vi "Ball Align(SubVI).vi"(0 "Align X - t, Y - f":bool, 2 "accuracy":u32=100, 3 "x is in range":bool, 4 "y is in range":bool, 5 "L_PWM":dbl=0.3, 6 "R_PWM":dbl=0.3, 7 "curX":dbl, 8 "defY":dbl, 9 "curY":dbl, 14 "defX":dbl, 16 "RangeY":dbl, 18 "RangeX":dbl=20.0) -> (13 "x_is_in_range":bool, 15 "y_is_in_range":bool, 19 "Ready to Grab()":bool, 20 "Align_X-t,Y-f":bool, 22 "accuracy out":u32=100, 26 "L_PWM out":dbl, 27 "R_PWM out":dbl)   [LabVIEW 2017]
uses:
  <vilib>/myRIO/Instrument Drivers/Onboard IO/DIO/typedefs/DIO Reference.ctl
  <vilib>/myRIO/Common/Instrument Driver Framework/Utilities/typedefs/myRIO Generic Hardware Reference.ctl
  <vilib>/myRIO/Common/Instrument Driver Framework/Utilities/typedefs/Hardware Version Enum.ctl
  <vilib>/myRIO/Common/Instrument Driver Framework/Utilities/typedefs/myRIO v1.0 Reference.ctl
  <vilib>/myRIO/Common/Instrument Driver Framework/Utilities/typedefs/Generic FPGA Reference.ctl
  <vilib>/myRIO/Common/Instrument Driver Framework/myRIO v1.0/DIO/typedefs/DIO Channels List.ctl
  <vilib>/myRIO/Common/Instrument Driver Framework/myRIO v1.0/DIO/typedefs/DIO Channels Enum.ctl
  <vilib>/userdefined/High Color/nirio_resource_hc.ctl
  <vilib>/myRIO/Common/Instrument Driver Framework/Utilities/vis/Is FPGA Ref Available.vi
  <vilib>/myRIO/Common/Instrument Driver Framework/myRIO v1.0/DIO/vis/myRIO v1.1 Open DIO.vi
  <vilib>/myRIO/Instrument Drivers/Onboard IO/DIO/vis/Write.vi
  <vilib>/myRIO/Common/Instrument Driver Framework/Utilities/vis/Validate Channels.vi
  <vilib>/myRIO/Common/Instrument Driver Framework/myRIO v1.0/DIO/vis/myRIO v1.0 Reserve DIO.vi
  <vilib>/myRIO/Common/Instrument Driver Framework/myRIO v1.0/Resource Manager/vis/myRIO v1.0 Reserve Channel List.vi
  <vilib>/myRIO/Common/Instrument Driver Framework/myRIO v1.0/DIO/vis/myRIO v1.0 Build MUX Configuration DIO.vi
  <vilib>/myRIO/Common/Instrument Driver Framework/myRIO v1.0/Resource Manager/vis/myRIO v1.0 Reserve Channel.vi
  <vilib>/myRIO/Common/Instrument Driver Framework/myRIO v1.0/Resource Manager/vis/myRIO v1.0 Unreserve Channel.vi
  <vilib>/myRIO/Common/Instrument Driver Framework/myRIO v1.0/Resource Manager/vis/myRIO v1.0 Create Configuration List.vi
  <vilib>/myRIO/Common/Instrument Driver Framework/myRIO v1.0/Resource Manager/vis/myRIO v1.0 Build Mutex Name.vi
  <vilib>/Utility/VariantDataType/GetNumericInfo.vi
  <vilib>/Utility/error.llb/Error Cluster From Error Code.vi
  <vilib>/myRIO/Common/Instrument Driver Framework/myRIO v1.0/myRIO v1.1 Open.vi
  <vilib>/myRIO/Common/Instrument Driver Framework/Utilities/vis/IO Manager.vi
  <vilib>/myRIO/Common/Instrument Driver Framework/Utilities/vis/Configuration Manager.vi
  <vilib>/myRIO/Common/Instrument Driver Framework/myRIO v1.0/Resource Manager/vis/myRIO v1.0 Configure IO.vi
  <vilib>/myRIO/Common/Instrument Driver Framework/myRIO v1.0/myRIO v1.0 Close.vi
  <vilib>/myRIO/Common/Instrument Driver Framework/myRIO v1.0/DIO/vis/myRIO v1.0 Write DIO.vi
  <vilib>/myRIO/Express VI/Onboard IO/DO/DO Express VI.xnode
  <vilib>/myRIO/Instrument Drivers/Onboard IO/DIO/vis/myRIO DIO Open.xnode
  <vilib>/myRIO/Instrument Drivers/Onboard IO/DIO/DIO.lvlib
panel:
  out "DEF R_PWM":dbl
  out "DEF L_PWM":dbl
  in  "extra power":dbl=0.2 format="%#_13g"
  in  "range for boost":dbl=250.0
  out "offset":bool
  in  "M_offsetX":dbl=30.0
  in  "M_defY":dbl=250.0
  out "Right+":bool
  out "Left-":bool
  out "Left+":bool
  out "Right-":bool
  # "IN"
  # "OUT"
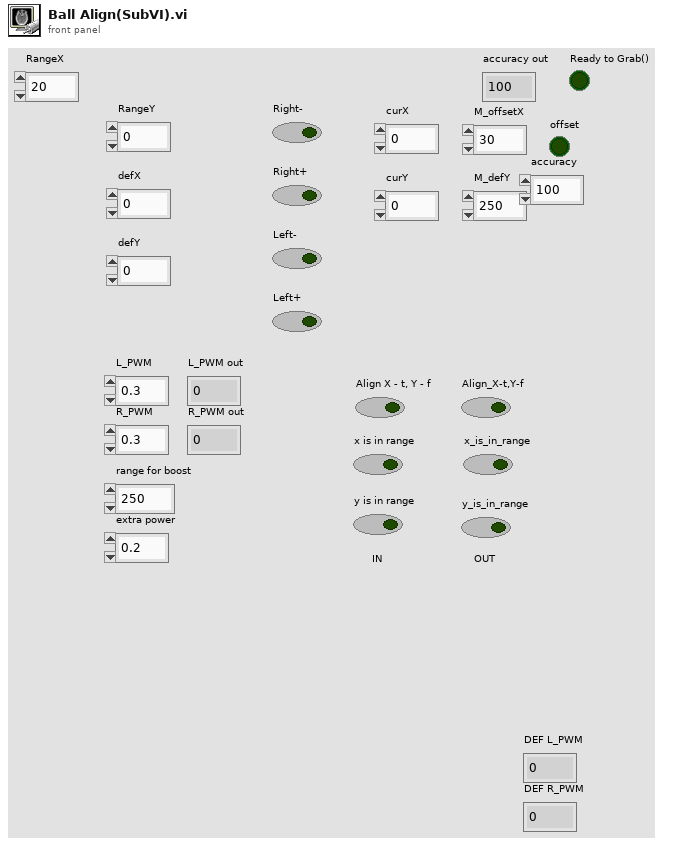
[diagram p1: front panel]
types:
  T1 = typedef "DIO.lvlib/DIO Reference.ctl" = cluster{"myRIO Reference":T2, "DIO Channels List":T6}
  T2 = typedef "myRIO Generic Hardware Reference.ctl" = cluster{"myRIO Model":T3, "myRIO Hardware Reference":T4}
  T3 = typedef "Hardware Version Enum.ctl" = enum16{"Unknown", "myRIO-1900", "myRIO-1950", "roboRIO", "NI ELVIS RIO CM"}
  T4 = typedef "myRIO v1.0 Reference.ctl" = cluster{"Generic FPGA Reference":T5, "Allow multiple opens":bool}
  T5 = typedef "Generic FPGA Reference.ctl" = refnum<k20>
  T6 = typedef "DIO Channels List.ctl" = T7[]
  T7 = typedef "DIO Channels Enum.ctl" = enum16{"Not Connected", "C/DIO0", "C/DIO1", "C/DIO2", "C/DIO3", "C/DIO4", "C/DIO5", "C/DIO6", "C/DIO7", "A/DIO0", "A/DIO1", "A/DIO2", "A/DIO3", "A/DIO4", "A/DIO5", "A/DIO6", "A/DIO7", "A/DIO8", "A/DIO9", "A/DIO10", "A/DIO11", "A/DIO12", "A/DIO13", "A/DIO14", "A/DIO15", "B/DIO0", "B/DIO1", "B/DIO2", "B/DIO3", "B/DIO4", "B/DIO5", "B/DIO6", "B/DIO7", "B/DIO8", "B/DIO9", "B/DIO10", "B/DIO11", "B/DIO12", "B/DIO13", "B/DIO14", "B/DIO15", "LED0", "LED1", "LED2", "LED3", "Button0", "DIO/DIO0", "DIO/DIO1", "DIO/DIO2", "DIO/DIO3", "DIO/DIO4", "DIO/DIO5", "DIO/DIO6", "DIO/DIO7", "DIO/DIO8", "DIO/DIO9", "SPI/CS0", "SPI/CS1", "SPI/CS2", "SPI/CS3", "LED RADIO (Green)", "LED RADIO (Red)", "LED COMM (Green)", "LED COMM (Red)", "LED MODE (Green)", "LED MODE (Red)"}
  T8 = typedef "nirio_resource_hc.ctl" = tag
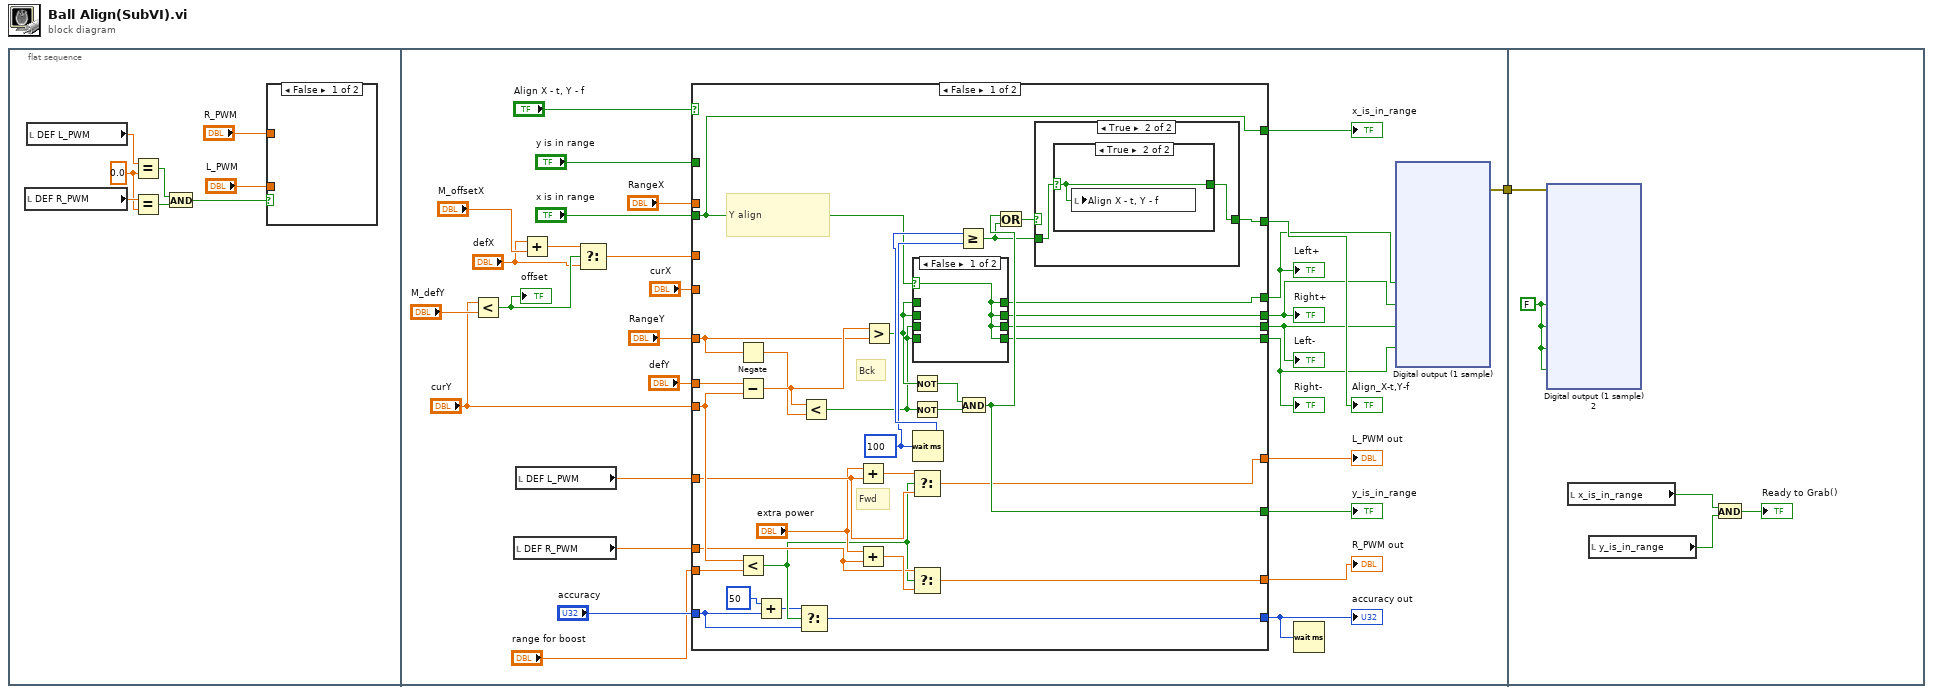
[diagram p0: block diagram]
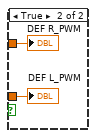
[diagram p2: hidden frame]
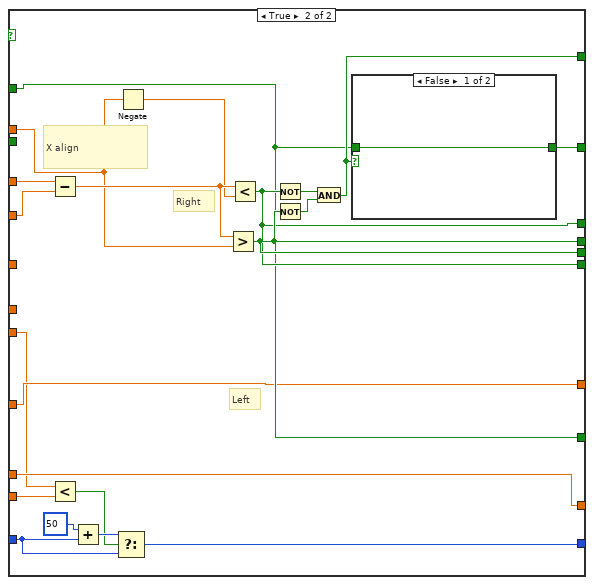
[diagram p6: hidden frame]
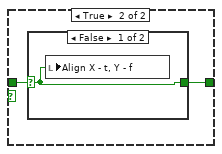
[diagram p7: hidden frame]
diagram:
  n1 = flat-sequence {
    tunnel: [w16] -> w1
    tunnel: w1 -> [w151]
    frame #0 {
      w2 = 0.0 ("y")
      n2 = local read "DEF R_PWM"() -> (w6:dbl)
      n3 = local read "DEF L_PWM"() -> (w5:dbl)
      n4 = Equal?(x=w5, y=w2) -> (x = y?=w8:bool)
      n5 = Equal?(x=w6, y=w2) -> (x = y?=w9:bool)
      n6 = And(x=w8, y=w9) -> (x .and. y?=w7:bool)
      n7 = case shown="False" w7 {
        tunnel: "L_PWM" -> [_ w11]
        tunnel: "R_PWM" -> [_ w10]
        frame False {
        }
        frame True {
          "DEF L_PWM" <- w11
          "DEF R_PWM" <- w10
        }
      }
    }
    frame #1 {
      n8 = Less?(x="curY", y="M_defY") -> (x < y?=w33:bool)
      "offset" <- w33
      n9 = local read "DEF R_PWM"() -> (w22:dbl)
      n10 = local read "DEF L_PWM"() -> (w21:dbl)
      n11 = Add(x="defX", y="M_offsetX") -> (x+y=w31:dbl)
      n12 = Select(t=w31, s=w33, f="defX") -> (s? t:f=w29:dbl)
      n13 = case shown="False" "Align X - t, Y - f" {
        tunnel: w29 -> [_ w138]
        tunnel: "curX" -> [_ w137]
        tunnel: "RangeY" -> [w108 _]
        tunnel: "defY" -> [w109 _]
        tunnel: "curY" -> [w99 w125]
        tunnel: [w107 w133] -> w39
        tunnel: [w91 w136] -> w40
        tunnel: [w88 w135] -> w12
        tunnel: [w89 w135] -> w15
        tunnel: [w87 w134] -> w13
        tunnel: [w90 w134] -> w14
        tunnel: "x is in range" -> [w91 _]
        tunnel: "y is in range" -> [_ w133]
        tunnel: [w100 w132] -> w25
        tunnel: w21 -> [w97 w130]
        tunnel: w22 -> [w94 w131]
        tunnel: [w93 w130] -> w24
        tunnel: [w92 w131] -> w23
        tunnel: "RangeX" -> [_ w129]
        tunnel: "accuracy" -> [w84 w123]
        tunnel: [w80 w122] -> w17
        tunnel: "range for boost" -> [w79 w126]
        frame False {
          w103 = u32 100 ("milliseconds to wait")
          # "Bck"
          # "Fwd"
          # "Y align"
          n14 = Negate(x=w108) -> (-x=w110:dbl)
          n15 = Subtract(x=w109, y=w99) -> (x-y=w111:dbl)
          n16 = Less?(x=w99, y=w79) -> (x < y?=w83:bool)
          n17 = Add(x=u32 50, y=w84) -> (x+y=w82:u32)
          n18 = Select(t=w82, s=w83, f=w84) -> (s? t:f=w80:u32)
          n19 = Less?(x=w111, y=w110) -> (x < y?=w85:bool)
          n20 = Add(x="extra power", y=w97) -> (x+y=w98:dbl)
          n21 = Add(x="extra power", y=w94) -> (x+y=w96:dbl)
          n22 = Greater?(x=w111, y=w108) -> (0:w86:bool)
          n23 = Not(x=w86) -> (.not. x?=w106:bool)
          n24 = Not(x=w85) -> (.not. x?=w105:bool)
          n25 = Select(t=w98, s=w83, f=w97) -> (s? t:f=w93:dbl)
          n26 = Select(t=w94, s=w83, f=w96) -> (s? t:f=w92:dbl)
          n27 = case shown="False" w91 {
            selector: w91 -> [w112 _]
            tunnel: [w112 w113] -> w90
            tunnel: w86 -> [_ w115]
            tunnel: w86 -> [_ w116]
            tunnel: [w112 w114] -> w89
            tunnel: w85 -> [_ w113]
            tunnel: [w112 w115] -> w88
            tunnel: w85 -> [_ w114]
            tunnel: [w112 w116] -> w87
            frame False {
            }
            frame True {
            }
          }
          n28 = Wait (ms)(milliseconds to wait=w103) -> (millisecond timer value=w104:u32)
          n29 = Greater Or Equal?(x=w104, y=w103) -> (x >= y?=w101:bool)
          n30 = And(x=w106, y=w105) -> (x .and. y?=w107:bool)
          n31 = Or(x=w107, y=w101) -> (x .or. y?=w102:bool)
          n32 = case shown="True" w102 {
            selector: w102 -> [w117 _]
            tunnel: w101 -> [_ w119]
            tunnel: [w117 w118] -> w100
            frame False {
            }
            frame True {
              n33 = case shown="True" w119 {
                selector: w119 -> [w120 w121]
                tunnel: [w120 w121] -> w118
                frame False {
                }
                frame True {
                  n34 = local write "Align X - t, Y - f"(w121) -> ()
                }
              }
            }
          }
        }
        frame True {
          # "X align"
          # "Right"
          # "Left"
          n35 = Subtract(x=w138, y=w137) -> (x-y=w142:dbl)
          n36 = Less?(x=w125, y=w126) -> (x < y?=w124:bool)
          n37 = Add(x=u32 50, y=w123) -> (x+y=w128:u32)
          n38 = Select(t=w128, s=w124, f=w123) -> (s? t:f=w122:u32)
          n39 = Negate(x=w129) -> (-x=w141:dbl)
          n40 = Greater?(x=w142, y=w129) -> (0:w135:bool)
          n41 = Less?(x=w142, y=w141) -> (x < y?=w134:bool)
          n42 = Not(x=w134) -> (.not. x?=w140:bool)
          n43 = Not(x=w135) -> (.not. x?=w139:bool)
          n44 = And(x=w140, y=w139) -> (x .and. y?=w136:bool)
          n45 = case shown="False" w136 {
            tunnel: w133 -> [w143 w145]
            tunnel: [w143 w144] -> w132
            frame False {
            }
            frame True {
              n46 = case shown="False" w145 {
                selector: w145 -> [w146 w147]
                tunnel: [w146 w147] -> w144
                frame False {
                  n47 = local write "Align X - t, Y - f"(w146) -> ()
                }
                frame True {
                }
              }
            }
          }
        }
      }
      "Right-" <- w14
      "Left+" <- w13
      "Left-" <- w15
      "Right+" <- w12
      "x_is_in_range" <- w40
      "y_is_in_range" <- w39
      "Align_X-t,Y-f" <- w25
      "L_PWM out" <- w24
      "R_PWM out" <- w23
      "accuracy out" <- w17
      n48 = Wait (ms)(milliseconds to wait=w17) -> ()  [unwired: 1 out]
      n49 = xnode "Digital output (1 sample)"("Left+ (A/DIO5 (Pin 21))"=w13, "Right+ (A/DIO7 (Pin 25))"=w12, "Left- (A/DIO6 (Pin 23))"=w15, "Right- (A/DIO13 (Pin 26))"=w14) -> ("error out"=w16:errorcluster)  [unwired: 1 in]
    }
    frame #2 {
      w152 = FALSE ("Left+ (A/DIO5 (Pin 21))")
      n50 = xnode "Digital output (1 sample) 2"("Left+ (A/DIO5 (Pin 21))"=w152, "Right+ (A/DIO7 (Pin 25))"=w152, "Left- (A/DIO6 (Pin 23))"=w152, "Right- (A/DIO13 (Pin 26))"=w152, "error in (no error)"=w151) -> ()  [unwired: 1 out]
      n51 = local read "x_is_in_range"() -> (w149:bool)
      n52 = local read "y_is_in_range"() -> (w150:bool)
      n53 = And(x=w149, y=w150) -> (x .and. y?=→"Ready to Grab()":bool)
    }
  }
